vi "KH TURCK Status AI Write.vi"(8 "TBEN-S2-4AI Input Values":T1) -> (3 "Status":bool[](array[boolean]))   [LabVIEW 2021]
uses:
  KH TURCK ETHERNETIP TDefCluster TBEN-S2-4AI Input Values.ctl
panel:
  # "Wire Break"
  # "upper limit"
  # "Overflow"
  # "Underflow"
  # "CJC Wire Break"
  # "Overcurrent (RTD)"
  # "Overcurrent supply VAUX1"
  # "Lower limit value underrun"
  # "Ch0"
  # "Ch1"
  # "Ch2"
  # "Ch3"
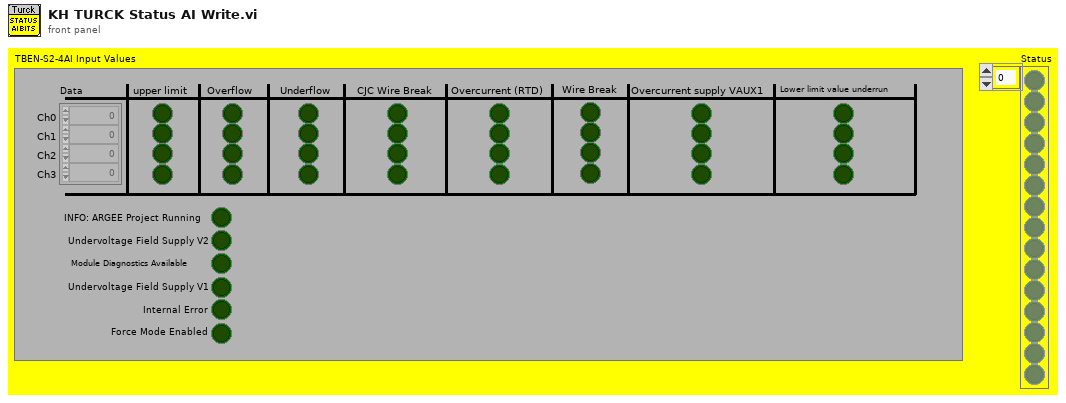
[diagram p1: front panel]
types:
  T1 = typedef "KH TURCK ETHERNETIP TDefCluster TBEN-S2-4AI Input Values.ctl" = cluster{"Data":i16[], "upper Limit CH0":bool, "upper Limit CH1":bool, "upper Limit CH2":bool, "upper Limit CH3":bool, "Overflow CH0":bool, "Overflow CH1":bool, "Overflow CH2":bool, "Overflow CH3":bool, "Underflow CH0":bool, "Underflow CH1":bool, "Underflow CH2":bool, "Underflow CH3":bool, "CJC Wire Break CH0":bool, "CJC Wire Break CH1":bool, "CJC Wire Break CH2":bool, "CJC Wire Break CH3":bool, "Overcurrent (RTD) CH0":bool, "Overcurrent (RTD) CH1":bool, "Overcurrent (RTD) CH2":bool, "Overcurrent (RTD) CH3":bool, "Wire Break CH0":bool, "Wire Break CH1":bool, "Wire Break CH2":bool, "Wire Break CH3":bool, "Overcurrent supply VAUX1 CH0":bool, "Overcurrent supply VAUX1 CH1":bool, "Overcurrent supply VAUX1 CH2":bool, "Overcurrent supply VAUX1 CH3":bool, "Lower limit value underrun CH0":bool, "Lower limit value underrun CH1":bool, "Lower limit value underrun CH2":bool, "Lower limit value underrun CH3":bool, "Module Diagnostics Available":bool, "INFO: ARGEE Project Running":bool, "Undervoltage Field Supply V2":bool, "Undervoltage Field Supply V1":bool, "Internal Error":bool, "Force Mode Enabled":bool}
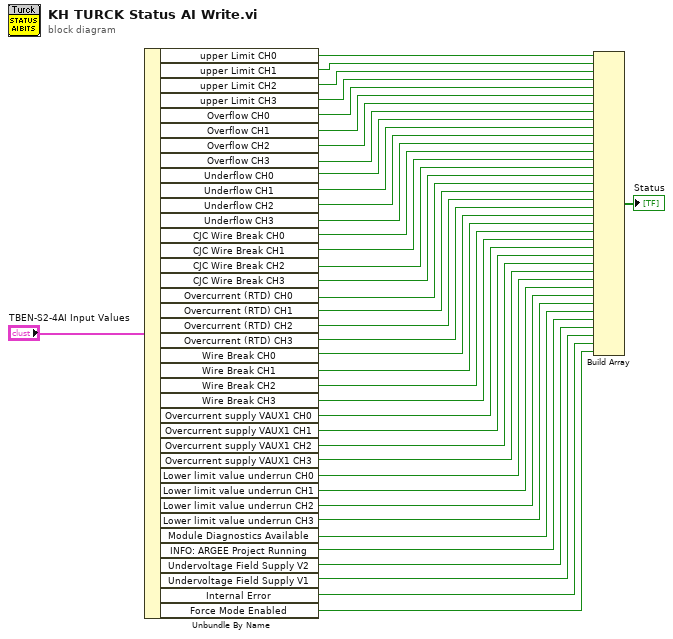
[diagram p0: block diagram]
diagram:
  n1 = Unbundle By Name("TBEN-S2-4AI Input Values") -> ("upper Limit CH0"=w39:bool, "upper Limit CH1"=w38:bool, "upper Limit CH2"=w37:bool, "upper Limit CH3"=w36:bool, "Overflow CH0"=w35:bool, "Overflow CH1"=w34:bool, "Overflow CH2"=w33:bool, "Overflow CH3"=w32:bool, "Underflow CH0"=w31:bool, "Underflow CH1"=w30:bool, "Underflow CH2"=w29:bool, "Underflow CH3"=w28:bool, "CJC Wire Break CH0"=w27:bool, "CJC Wire Break CH1"=w26:bool, "CJC Wire Break CH2"=w25:bool, "CJC Wire Break CH3"=w24:bool, "Overcurrent (RTD) CH0"=w23:bool, "Overcurrent (RTD) CH1"=w22:bool, "Overcurrent (RTD) CH2"=w21:bool, "Overcurrent (RTD) CH3"=w20:bool, "Wire Break CH0"=w19:bool, "Wire Break CH1"=w18:bool, "Wire Break CH2"=w17:bool, "Wire Break CH3"=w16:bool, "Overcurrent supply VAUX1 CH0"=w15:bool, "Overcurrent supply VAUX1 CH1"=w14:bool, "Overcurrent supply VAUX1 CH2"=w13:bool, "Overcurrent supply VAUX1 CH3"=w12:bool, "Lower limit value underrun CH0"=w11:bool, "Lower limit value underrun CH1"=w10:bool, "Lower limit value underrun CH2"=w9:bool, "Lower limit value underrun CH3"=w8:bool, "Module Diagnostics Available"=w7:bool, "INFO: ARGEE Project Running"=w6:bool, "Undervoltage Field Supply V2"=w5:bool, "Undervoltage Field Supply V1"=w4:bool, "Internal Error"=w3:bool, "Force Mode Enabled"=w2:bool)
  n2 = Build Array(w39, w38, w37, w36, w35, w34, w33, w32, w31, w30, w29, w28, w27, w26, w25, w24, w23, w22, w21, w20, w19, w18, w17, w16, w15, w14, w13, w12, w11, w10, w9, w8, w7, w6, w5, w4, w3, w2) -> (→"Status":bool[])
